vi "calc_lorentzian.vi"(9 "Width in":dbl, 10 "x in":dbl, 11 "Position in":dbl) -> (3 "Value out":dbl)   [LabVIEW 2018]
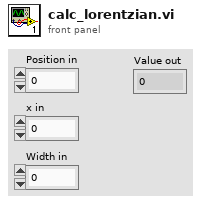
[diagram p1: front panel]
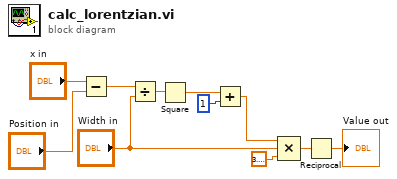
[diagram p0: block diagram]
diagram:
  n1 = Subtract(x="x in", y="Position in") -> (x-y=w8:dbl)
  n2 = Divide(x=w8, y="Width in") -> (x/y=w7:dbl)
  n3 = Square(x=w7) -> (x^2=w5:dbl)
  n4 = Add(x=w5, y=1) -> (x+y=w4:dbl)
  n5 = Compound Arithmetic op=MULTIPLY(w4, "Width in", 3.141592653589793) -> (w1:dbl)
  n6 = Reciprocal(x=w1) -> (1/x=→"Value out":dbl)
